vi "Flatten Variant Bitness.vi"(8 "error in (no error)":errorcluster, 9 "byte order (0:big-endian, network order)":T1(ring), 10 "Prepend Array or String size (T)":bool=TRUE, 11 "Variant":variant) -> (0 "error out":errorcluster, 3 "data string":string)   [LabVIEW 2020, in "LV Tiff.lvlib"]
uses:
  LV Tiff.lvlib
  <vilib>/Utility/Data Type/NI_Data Type.lvlib
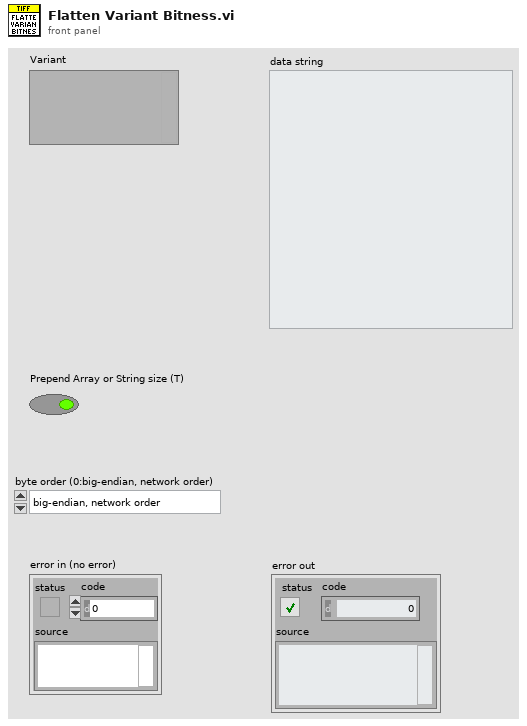
[diagram p1: front panel]
types:
  T1 = enum16{"big-endian, network order", "native, host order", "little-endian"}
  T2 = typedef "NI_Data Type.lvlib/Data Type.ctl" = enum8{"Invalid Type", "Void", "I8", "I16", "I32", "I64", "U8", "U16", "U32", "U64", "Single Float", "Double Float", "Extended Float", "Single Complex", "Double Complex", "Extended Complex", "Enum U8", "Enum U16", "Enum U32", "Enum U64", "Single Float With Unit", "Double Float With Unit", "Extended Float With Unit", "Single Complex with Unit", "Double Complex with Unit", "Extended Complex with Unit", "Boolean", "String", "Path", "Picture", "Tag", "Array", "Cluster", "Variant", "LV Variant", "Waveform", "Timestamp", "Digital Waveform", "Digital Data", "ExpressData", "Refnum", "External Data", "VI", "Poly VI", "LabVIEW Class Instance", "Fixed Point", "Set Collection", "Map Collection"}
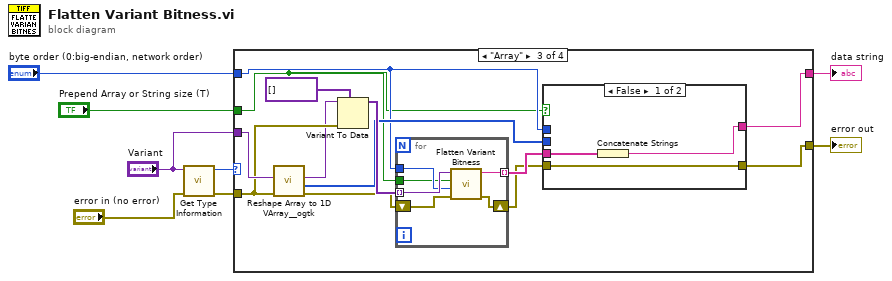
[diagram p0: block diagram]
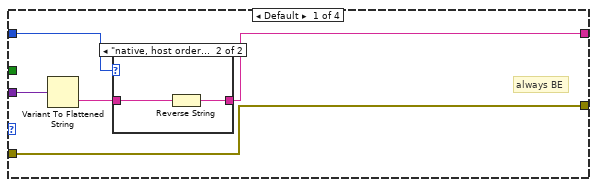
[diagram p2: hidden frame]
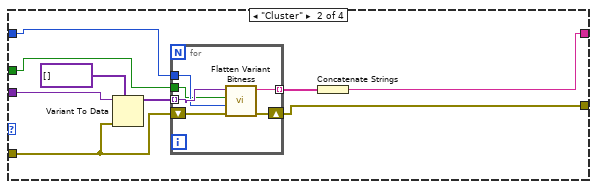
[diagram p4: hidden frame]
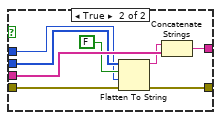
[diagram p5: hidden frame]
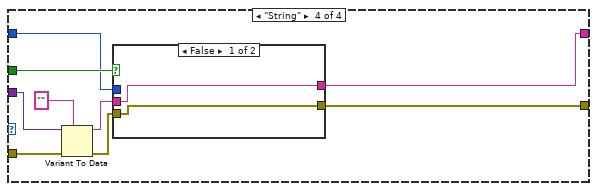
[diagram p6: hidden frame]
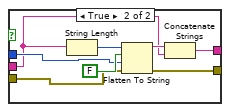
[diagram p7: hidden frame]
diagram:
  n1 = call <vilib>:"Get Type Information.vi"("error in (no error)"="error in (no error)", "variant"="Variant") -> ("error out"=w4:errorcluster, "type"=w7:T2)  [unwired: 5 in, 3 out]
  n2 = case shown="\"Array\"" w7 {
    tunnel: "Variant" -> [w13 w25 w40 w70]
    tunnel: [w10 w20 w41 w66] -> w6
    tunnel: "byte order (0:big-endian, network order)" -> [w12 w22 w37 w64]
    tunnel: w4 -> [w9 w18 w39 w68]
    tunnel: "Prepend Array or String size (T)" -> [_ w19 w36 w67]
    tunnel: [w9 w17 w34 w62] -> w1
    frame Default {
      # "always BE"
      n3 = Variant To Flattened String(Variant=w13) -> (data string=w11:string)  [unwired: 1 out]
      n4 = case shown="\"native, host order\", \"little-endian\"" w12 {
        tunnel: w11 -> [w14 w16]
        tunnel: [w14 w15] -> w10
        frame "big-endian, network order", Default {
        }
        frame "native, host order", "little-endian" {
          n5 = Reverse String(1:w16) -> (0:w15:string)
        }
      }
    }
    frame "Cluster" {
      n6 = Variant To Data(error in=w18, type=variant[] [], Variant=w25) -> (data=w23:variant[])  [unwired: 1 out]
      n7 = for {
        tunnel: w23 -> [w31] mode=indexing
        tunnel: w22 -> [w30]
        tunnel: [w29] -> w21 mode=indexing
        tunnel: w19 -> [w28]
        shift-right: [w26] -> w17
        shift-left: w18 -> [w27]
        n8 = call "Flatten Variant Bitness.vi"("error in (no error)"=w27, "byte order (0:big-endian, network order)"=w30, "Prepend Array or String size (T)"=w28, "Variant"=w31) -> ("error out"=w26:errorcluster, "data string"=w29:string)  [unwired: 6 in]
      }
      n9 = Concatenate Strings(w21) -> (w20:string)
    }
    frame "Array" {
      n10 = call <userlib>:"Reshape Array to 1D VArray__ogtk.vi"("error in (no error)"=w39, "MultiD Array"=w40) -> ("error out"=w33:errorcluster, "Size(s)"=w38:u32[], "1D VArray"=w35:variant)  [unwired: 7 in]
      n11 = Variant To Data(error in=w39, type=variant[] [], Variant=w35) -> (data=w43:variant[])  [unwired: 1 out]
      n12 = for {
        tunnel: w43 -> [w61] mode=indexing
        tunnel: w37 -> [w60]
        tunnel: [w59] -> w42 mode=indexing
        tunnel: w36 -> [w58]
        shift-right: [w56] -> w32
        shift-left: w33 -> [w57]
        n13 = call "Flatten Variant Bitness.vi"("error in (no error)"=w57, "byte order (0:big-endian, network order)"=w60, "Prepend Array or String size (T)"=w58, "Variant"=w61) -> ("error out"=w56:errorcluster, "data string"=w59:string)  [unwired: 6 in]
      }
      n14 = case shown="False" w36 {
        tunnel: w42 -> [w47 w55]
        tunnel: [w46 w54] -> w41
        tunnel: w38 -> [_ w53]
        tunnel: w37 -> [_ w51]
        tunnel: w32 -> [w45 w50]
        tunnel: [w45 w48] -> w34
        frame False {
          n15 = Concatenate Strings(w47) -> (w46:string)
        }
        frame True {
          n16 = Flatten To String(anything=w53, prepend array or string size? (T)=FALSE, byte order (0:big-endian, network order)=w51, error in (no error)=w50) -> (data string=w49:string, error out=w48:errorcluster)  [unwired: 1 out]
          n17 = Concatenate Strings(w49, w55) -> (w54:string)
        }
      }
    }
    frame "String" {
      n18 = Variant To Data(error in=w68, type="", Variant=w70) -> (data=w65:string, error out=w63:errorcluster)
      n19 = case shown="False" w67 {
        tunnel: [w72 w74] -> w66
        tunnel: w65 -> [w72 w75]
        tunnel: w64 -> [_ w78]
        tunnel: w63 -> [w71 w77]
        tunnel: [w71 w73] -> w62
        frame False {
        }
        frame True {
          n20 = String Length(string=w75) -> (length=w80:i32)
          n21 = Flatten To String(anything=w80, prepend array or string size? (T)=FALSE, byte order (0:big-endian, network order)=w78, error in (no error)=w77) -> (data string=w76:string, error out=w73:errorcluster)  [unwired: 1 out]
          n22 = Concatenate Strings(w76, w75) -> (w74:string)
        }
      }
    }
  }
  "data string" <- w6
  "error out" <- w1
